vi "Make start scan activity string.vi"(11 "Sample ID":string) -> (3 "Array":T1[](array[typedef]) {"Epoch sec" format="%.2e"})   [LabVIEW 2013]
uses:
  User Access Type defs/Acitivity cluster.ctl
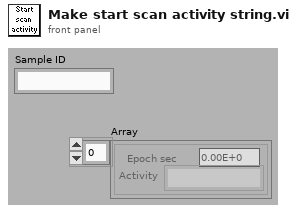
[diagram p1: front panel]
types:
  T1 = typedef "Acitivity cluster.ctl" = cluster{"Epoch sec":dbl, "Activity":string}
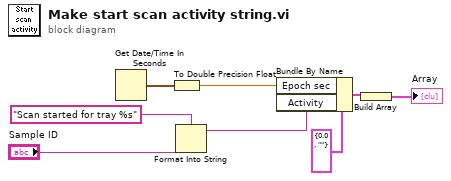
[diagram p0: block diagram]
diagram:
  n1 = Get Date/Time In Seconds() -> (seconds since 1Jan1904=w4:timestamp)
  n2 = To Double Precision Float(number=w4) -> (double precision float=w5:dbl)
  n3 = Format Into String(format string="Scan started for tray %s" ("Activity"), "Sample ID") -> (resulting string=w1:string)  [unwired: 2 in, 1 out]
  n4 = Bundle By Name(cluster=T1 {"Epoch sec"=0.0, "Activity"=""} ("Cluster"), "Epoch sec"=w5, "Activity"=w1) -> (w7:T1)
  n5 = Build Array(w7) -> (→"Array":T1[])
